vi "Demo.vi"() -> ()   [LabVIEW 2020]
uses:
  BlingLibrary/WriteLedArrayStatus.ctl
  <vilib>/Platform/TimedLoop/XDataNode/timing_clust.ctl
  <vilib>/Platform/TimedLoop/XDataNode/nitl_modes.ctl
  <vilib>/Platform/TimedLoop/XDataNode/wakeup.ctl
  <vilib>/platform/TimedLoop/XDataNode/XDataNode.xnode
  BlingLibrary/ArduinoSerialBling.lvlib
  <vilib>/Platform/TimedLoop/XDataNode/XDNodeRunTimeDep.lvlib
panel:
  in  "Chain Setup":cluster{"ChainNumber":u8, "numLeds":u8}[](array[cluster])=[{"ChainNumber"=0, "numLeds"=150}]
  in  "OfflineMode":bool
  out "Colors":u32[](array[colorbox])
  out "Write Array Status":T1
  out "Frequency":dbl(graph)
  in  "Value Width":enum16{"4-bit", "8-bit"}(ring)
  in  "Reset on open?":bool=TRUE
  in  "Synchronous":bool=TRUE
  out "Loops":i32
  in  "Sine Rate":i32=50
  in  "Tab Control":T2(tab)
  in  "Period":i32=200
  in  "Color 2":u32(colorbox)=16860
  in  "Color 1":u32(colorbox)=16711680
  in  "Period (ms)":i32=500
  in  "Color 2":u32(colorbox)
  in  "Color 1":u32(colorbox)=16711680
  in  "Color":u32(colorbox)
  in  "MaxColor":u32(colorbox)=16448250
  in  "Color Box":u32(colorbox)=16711680
  in  "Color 1":u32(colorbox)=16711680
  in  "Color 2":u32(colorbox)=16860
  in  "Colors":u32[](array[colorbox])
  in  "Background Color":u32(colorbox)
  in  "Foreground Color":u32(colorbox)=16711680
  in  "Blending LEDs":u8=10
  in  "stop":bool
  in  "Serial Port":refnum<visa-resource-name>
  # "Options to set prior to run"
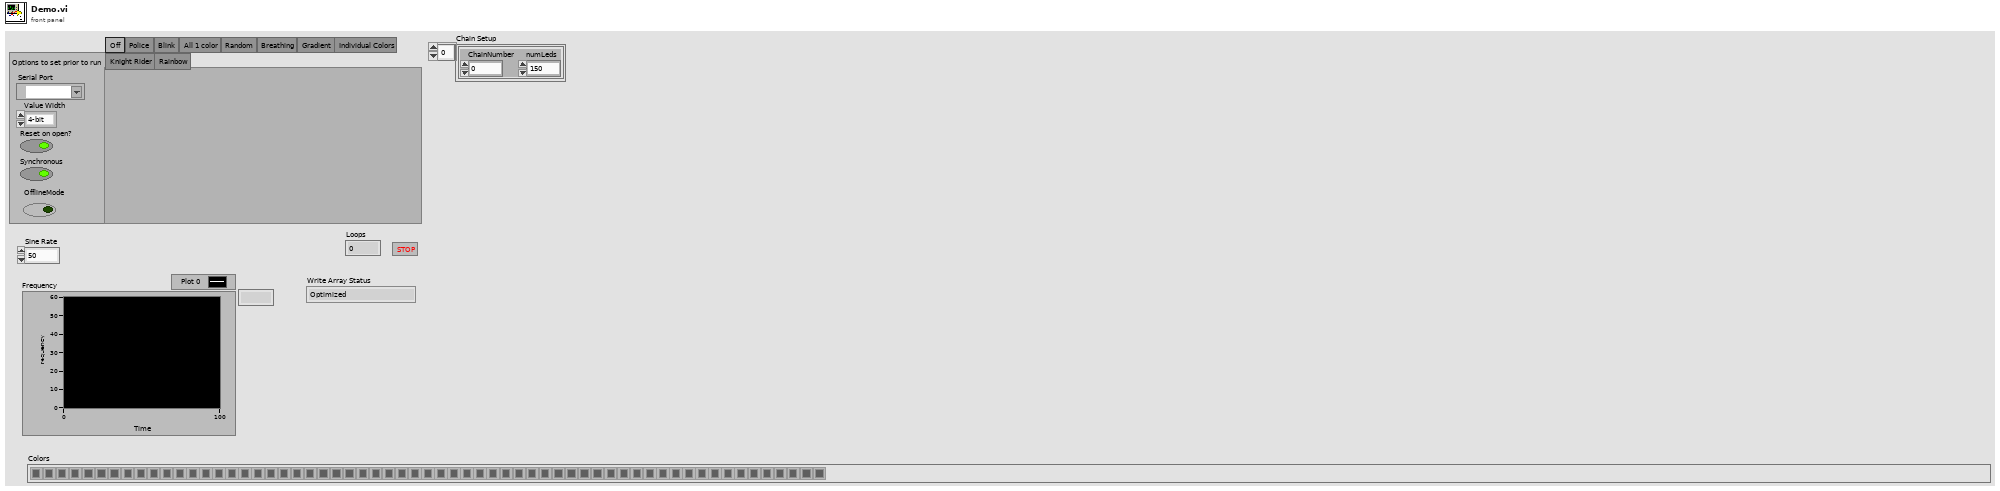
[diagram p1: front panel]
types:
  T1 = typedef "ArduinoSerialBling.lvlib/WriteLedArrayStatus.ctl" = enum16{"Optimized", "Unable to optimize", "No changes", "Error", "Offline"}
  T2 = enum32{"Off", "Police", "Blink", "All 1 color", "Random", "Breathing", "Gradient", "Individual Colors", "Knight Rider", "Rainbow"}
  T3 = typedef "ArduinoSerialBling.lvlib/ControlState.ctl" = cluster{"VISA resource name":refnum<visa-resource-name>, "Synchronous":bool, "Value Width":enum16{"4-bit", "8-bit"}, "ChainMask":u8, "Chains":T4[], "OfflineMode":bool}
  T4 = typedef "ArduinoSerialBling.lvlib/ChainState.ctl" = cluster{"ChainNumber":u8, "numLeds":u8, "LED Colors":u32[]}
  T5 = typedef "XDNodeRunTimeDep.lvlib/timing_clust.ctl" = cluster{"Expected End [f-1]":u64, "Actual End [f-1]":u64, "Finished Late? [f-1]":bool, "Expected End [i-1]":u64, "Actual End [i-1]":u64, "Finished Late? [i-1]":bool, "Expected Start [i]":u64, "Actual Start [i]":u64, "Expected Start [f]":u64, "Actual Start [f]":u64, "Source Name":string, "Structure Name":string, "Period":i64, "Deadline":i64, "Offset":i64, "Start":i64, "Priority":i32, "Timeout":i32, "Mode":T6, "Wakeup Reason":T7, "Error":errorcluster, "Source Type":string, "Secondary Source Type":string, "Global End Time":u64, "Global Start Time":u64, "Frame Duration":u64, "Iteration Duration":u64, "Assigned CPU":i32, "I/O Scan Engine Mode":u32}
  T6 = typedef "XDNodeRunTimeDep.lvlib/nitl_modes.ctl" = enum32{"No Change", "Process missed periods, maintain original phase", "Discard missed periods, maintain original phase", "Process missed periods, ignore original phase", "Discard missed periods, ignore original phase"}
  T7 = typedef "XDNodeRunTimeDep.lvlib/wakeup.ctl" = enum32{"Normal", "Aborted", "Asynchronous wakeup", "Timing source error", "Timed loop error", "Timeout"}
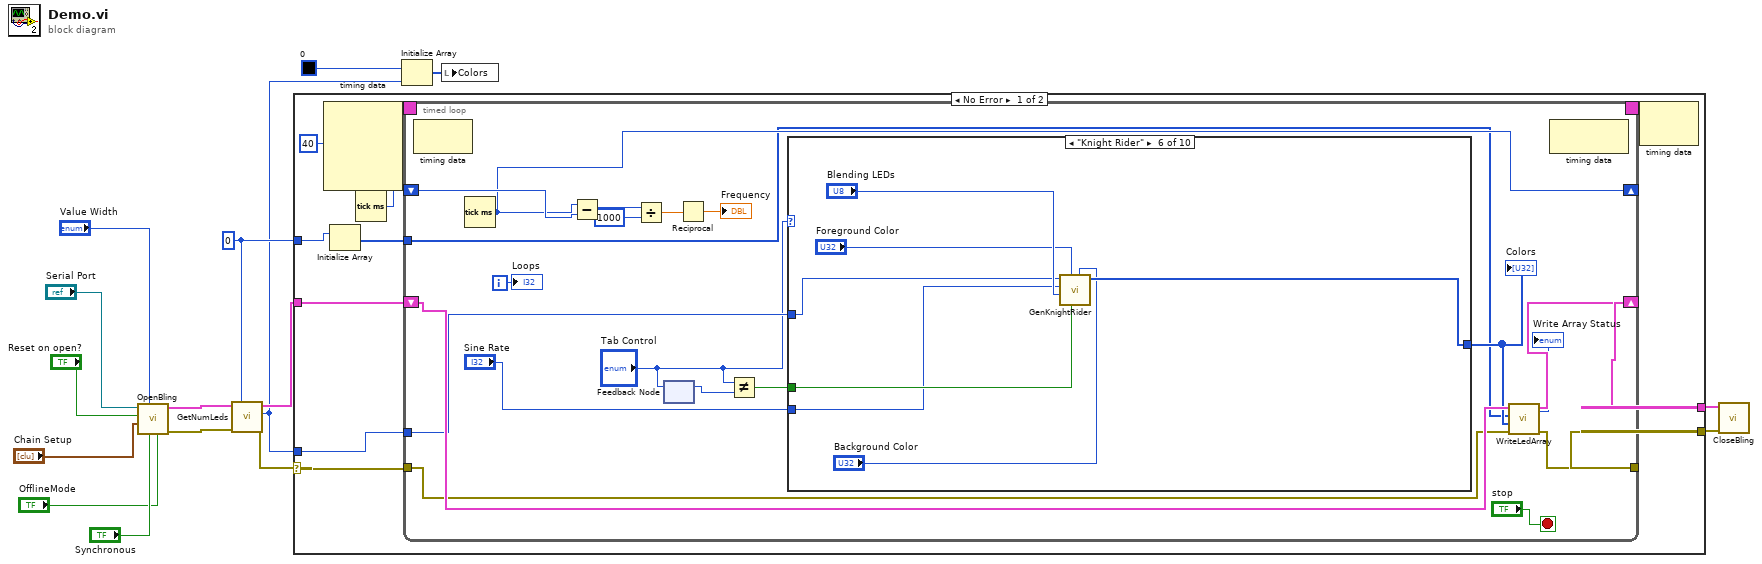
[diagram p0: block diagram]
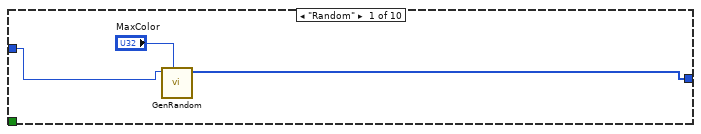
[diagram p2: hidden frame]
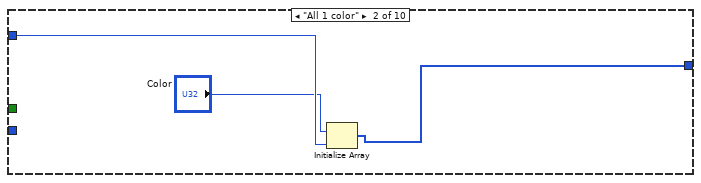
[diagram p3: hidden frame]
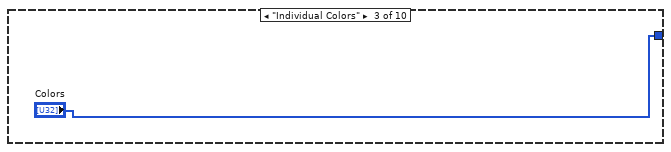
[diagram p4: hidden frame]
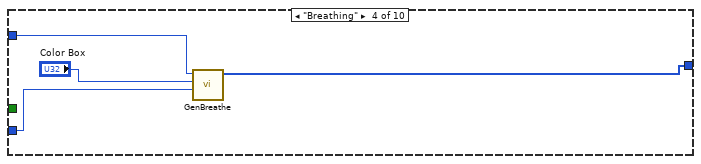
[diagram p5: hidden frame]
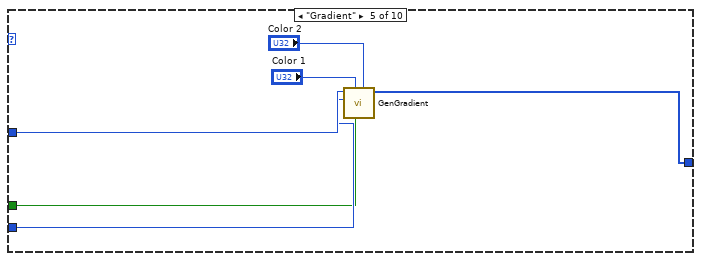
[diagram p6: hidden frame]
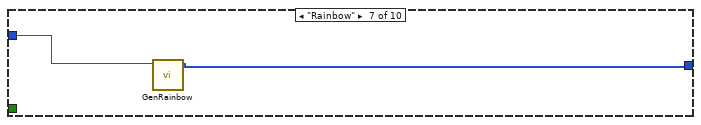
[diagram p7: hidden frame]
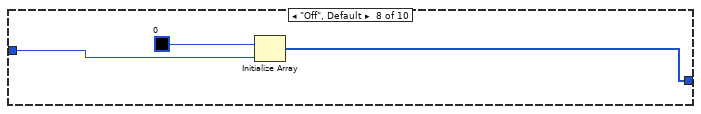
[diagram p8: hidden frame]
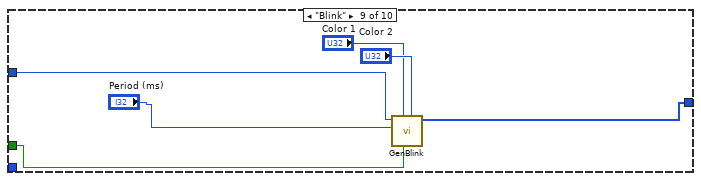
[diagram p9: hidden frame]
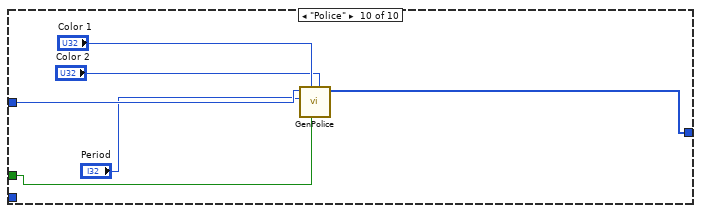
[diagram p10: hidden frame]
diagram:
  w7 = 0
  n1 = call "OpenBling.vi"("OfflineMode"="OfflineMode", "Synchronous"="Synchronous", "Value Width"="Value Width", "Chain Setup"="Chain Setup", "Reset on open?"="Reset on open?", "Serial Port"="Serial Port") -> ("error out"=w8:errorcluster, "ControlState"=w9:T3)  [unwired: 4 in]
  n2 = call "GetNumLeds.vi"("error in (no error)"=w8, "Chain"=w7, "ControlState"=w9) -> ("error out"=w4:errorcluster, "NumLeds"=w1:i32, "ControlState 2"=w6:T3)  [unwired: 6 in]
  n3 = case shown="No Error" w4 {
    selector: w4 -> [w23 w95]
    tunnel: [w27 w95] -> w13
    tunnel: [w26 w96] -> w12
    tunnel: w7 -> [w17 _]
    tunnel: w6 -> [w25 w96]
    tunnel: w1 -> [w24 _]
    frame No Error {
      n4 = node-c288(i64 40 ("Period")) -> (w21:T5)  [unwired: 3 in]
      n5 = Initialize Array(w17) -> (w18:i32[])  [unwired: 1 in]
      n6 = Tick Count (ms)() -> (millisecond timer value=w22:u32)
      n7 = timed-loop {
        tunnel: w18 -> [w28]
        tunnel: w24 -> [w33]
        tunnel: w23 -> [w46]
        tunnel: [w37] -> w27
        shift-right: [w43] -> _
        shift-left: w22 -> [w44]
        shift-right: [w36] -> w26
        shift-left: w25 -> [w47]
        timing: w21 -> [_]
        timing-out: [_] -> w20
        i -> [w34]
        stop <- "stop" stop-if-true
        n8 = node-c288() -> ()  [unwired: 1 in, 1 out]
        n9 = Tick Count (ms)() -> (millisecond timer value=w43:u32)
        n10 = Subtract(x=w43, y=w44) -> (x-y=w42:u32)
        n11 = Divide(x=w42, y=u32 1000) -> (x/y=w40:dbl)
        n12 = feedback-in #1("Tab Control") -> ()
        n13 = feedback #1() -> (w31:T2)  [unwired: 1 in]
        n14 = Reciprocal(x=w40) -> (1/x=→"Frequency":dbl)
        n15 = Not Equal?(x="Tab Control", y=w31) -> (x != y?=w30:bool)
        n16 = case shown="\"Knight Rider\"" "Tab Control" {
          tunnel: w33 -> [w50 w55 _ w59 w63 w68 w75 w77 w80 w86]
          tunnel: "Sine Rate" -> [_ _ _ w57 w62 w67 _ _ _ _]
          tunnel: [w52 w54 "Colors" w58 w66 w73 w74 w76 w83 w89] -> w38
          tunnel: w30 -> [_ _ _ _ w61 w71 _ _ w84 w90]
          frame "Random" {
            n17 = call "GenRandom.vi"("MaxColor"="MaxColor", "NumLeds"=w50) -> ("Array"=w52:u32[])  [unwired: 9 in]
          }
          frame "All 1 color" {
            n18 = Initialize Array("Color", w55) -> (w54:u32[])
          }
          frame "Individual Colors" {
          }
          frame "Breathing" {
            n19 = call "GenBreathe.vi"("Sine Rate"=w57, "Color Box"="Color Box", "NumLeds"=w59) -> ("Array"=w58:u32[])  [unwired: 7 in, 1 out]
          }
          frame "Gradient" {
            n20 = call "GenGradient.vi"("Color 2"="Color 2", "Reset"=w61, "Color 1"="Color 1", "Sine Rate"=w62, "NumLeds"=w63) -> ("LED Array"=w66:u32[])  [unwired: 6 in]
          }
          frame "Knight Rider" {
            n21 = call "GenKnightRider.vi"("Background Color"="Background Color", "Reset"=w71, "Foreground Color"="Foreground Color", "Blending LEDs"="Blending LEDs", "Sine Rate"=w67, "NumLeds"=w68) -> ("Array"=w73:u32[])  [unwired: 4 in, 1 out]
          }
          frame "Rainbow" {
            n22 = call "GenRainbow.vi"("NumLeds"=w75) -> ("Rainbow"=w74:u32[])  [unwired: 10 in]
          }
          frame "Off", Default {
            n23 = Initialize Array(u32 0 ("new element/subarray"), w77) -> (w76:u32[])
          }
          frame "Blink" {
            n24 = call "GenBlink.vi"("Color 2"="Color 2", "Reset"=w84, "Color 1"="Color 1", "Period (ms)"="Period (ms)", "NumLeds"=w80) -> ("Array"=w83:u32[])  [unwired: 5 in, 1 out]
          }
          frame "Police" {
            n25 = call "GenPolice.vi"("Color 2"="Color 2", "Reset"=w90, "Color 1"="Color 1", "Period"="Period", "NumLeds"=w86) -> ("Array"=w89:u32[])  [unwired: 6 in]
          }
        }
        "Colors" <- w38
        n26 = call "WriteLedArray.vi"("error in (no error)"=w46, "LED Colors"=w38, "Chains"=w28, "ControlState in"=w47) -> ("error out"=w37:errorcluster, "ControlState out"=w36:T3, "Optimization"=→"Write Array Status":T1)  [unwired: 5 in]
        n27 = node-c288() -> ()  [unwired: 1 in, 1 out]
        "Loops" <- w34
      }
      n28 = node-c288(w20) -> ()  [unwired: 1 out]
    }
    frame Error {
    }
  }
  n29 = Initialize Array(u32 0 ("new element/subarray"), w1) -> (w5:u32[])
  n30 = local write "Colors"(w5) -> ()
  n31 = call "CloseBling.vi"("error in (no error)"=w13, "ControlState in"=w12) -> ()  [unwired: 9 in, 1 out]
